vi "Read All Metrics.vi"(8 "error in (no error)":errorcluster, 11 "Default Collector in":refnum<class "Default Collector.lvclass">) -> (0 "error out":errorcluster, 2 "Metrics":refnum<data-value>[](array[refnum]), 3 "Default Collector out":refnum<class "Default Collector.lvclass">)   [LabVIEW 2020, in "Collector.lvlib" / "Default Collector.lvclass"]
uses:
  metrics/metric/Metric.lvclass
  Default Collector.lvclass
  Default Collector.lvclass/Default Collector.ctl
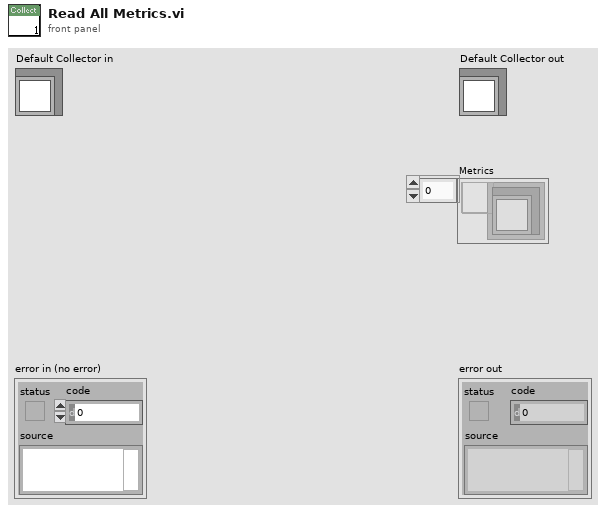
[diagram p1: front panel]
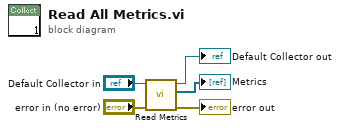
[diagram p0: block diagram]
diagram:
  n1 = call-dynamic "Read Metrics.vi"("error in (no error)"="error in (no error)", "Default Collector in"="Default Collector in") -> ("error out"=→"error out":errorcluster, "Metrics"=→"Metrics":refnum<data-value>[], "Default Collector out"=→"Default Collector out":refnum<class "Default Collector.lvclass">)  [unwired: 7 in]
